vi "Append Properties to Edit Context Menu.vi"(9 "State":T1={"Update"=FALSE, "Show advanced"=FALSE, "Fs (Hz)"=100000.0, "Show persist"=FALSE}, 11 "Menu in":refnum<k9>) -> ()   [LabVIEW 2020, in "Stimulus Channel (Full).xctl"]
uses:
  Stimulus Channel (Full).xctl
  State.ctl
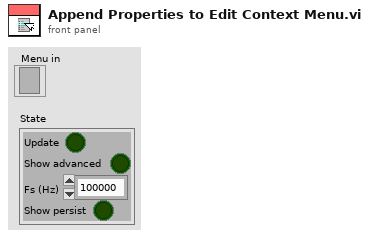
[diagram p1: front panel]
types:
  T1 = typedef "Stimulus Channel (Full).xctl/State.ctl" = cluster{"Update":bool, "Show advanced":bool, "Fs (Hz)":dbl, "Show persist":bool}
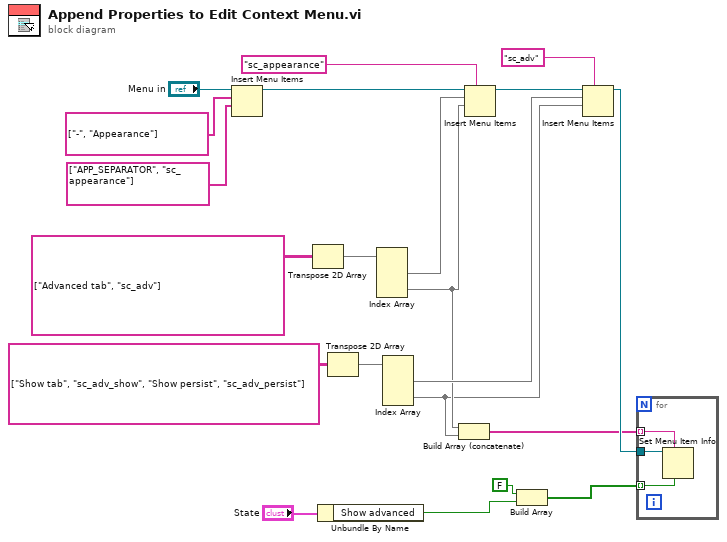
[diagram p0: block diagram]
diagram:
  n1 = Insert Menu Items(7:string[] ["APP_SEPARATOR", "sc_appearance"] ("item names"), 8:string[] ["-", "Appearance"] ("item names"), 9:"Menu in") -> (3:w20:refnum<k9>)  [unwired: 3 in, 2 out]
  n2 = Transpose 2D Array(2D array=string[][] [["Advanced tab", "sc_adv"]] ("item names")) -> (transposed array=w15:string[][])
  n3 = Unbundle By Name("State") -> ("Show advanced"=w5:bool)
  n4 = Transpose 2D Array(2D array=string[][] [["Show tab", "sc_adv_show"], ["Show persist", "sc_adv_persist"]] ("item names")) -> (transposed array=w10:string[][])
  n5 = Index Array(array=w15) -> (element #1=w14:string[], element #2=w7:string[])  [unwired: 4 in]
  n6 = Index Array(array=w10) -> (element #1=w9:string[], element #2=w6:string[])  [unwired: 4 in]
  n7 = Build Array (concatenate)(w7, w6) -> (w2:string[])
  n8 = Insert Menu Items(5:"sc_appearance", 7:w7, 8:w14, 9:w20) -> (3:w12:refnum<k9>)  [unwired: 2 in, 2 out]
  n9 = Build Array(FALSE ("element"), w5) -> (w3:bool[])
  n10 = Insert Menu Items(5:"sc_adv", 7:w6, 8:w9, 9:w12) -> (3:w4:refnum<k9>)  [unwired: 2 in, 2 out]
  n11 = for {
    tunnel: w4 -> [w24]
    tunnel: w3 -> [w23] mode=indexing
    tunnel: w2 -> [w22] mode=indexing
    n12 = Set Menu Item Info(6:w23, 7:w22, 11:w24) -> ()  [unwired: 4 in, 2 out]
  }
